vi "FGV_MG_Voltage_PCC.vi"(6 "Buffer Size":i32=10000, 7 "Command":T1, 8 "error in (no error)":errorcluster, 11 "Vabc":sgl[](array[numeric])) -> (0 "error out":errorcluster, 3 "Buffer":sgl[][](array[numeric]), 5 "Buffer Index":i32)   [LabVIEW 2015]
uses:
  Data_Queue_Command.ctl
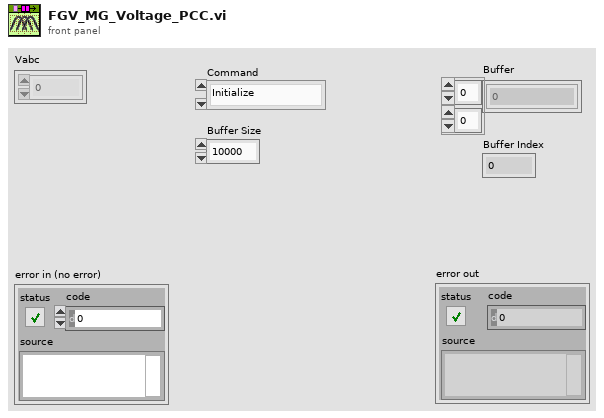
[diagram p1: front panel]
types:
  T1 = typedef "Data_Queue_Command.ctl" = enum16{"Initialize", "Write Sample", "Pull Array", "Close"}
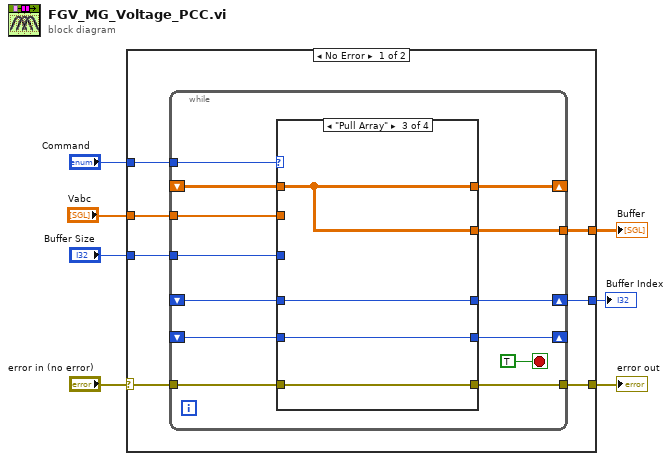
[diagram p0: block diagram]
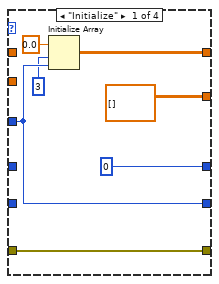
[diagram p2: hidden frame]
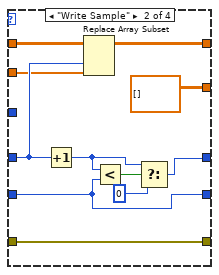
[diagram p3: hidden frame]
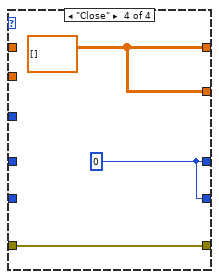
[diagram p4: hidden frame]
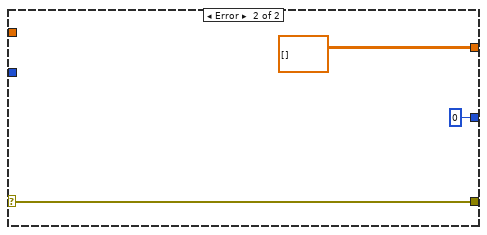
[diagram p5: hidden frame]
diagram:
  n1 = case shown="No Error" "error in (no error)" {
    selector: "error in (no error)" -> [w10 w55]
    tunnel: [w9 w55] -> w6
    tunnel: "Command" -> [w14 _]
    tunnel: "Buffer Size" -> [w13 _]
    tunnel: "Vabc" -> [w12 _]
    tunnel: [w11 sgl[][] []] -> w3
    tunnel: [w8 0 ("f")] -> w1
    frame No Error {
      n2 = while {
        tunnel: w14 -> [w26]
        tunnel: w13 -> [w25]
        tunnel: w12 -> [w24]
        shift-right: [w23] -> _
        shift-left: _ -> [w22]
        shift-right: [w21] -> _
        shift-left: _ -> [w20]
        shift-right: [w19] -> w8
        shift-left: _ -> [w18]
        tunnel: [w17] -> w11
        tunnel: w10 -> [w16]
        tunnel: [w15] -> w9
        stop <- TRUE stop-if-true
        n3 = case shown="\"Pull Array\"" w26 {
          tunnel: w25 -> [w29 _ _ _]
          tunnel: w24 -> [_ w35 _ _]
          tunnel: [w34 w40 w47 w52] -> w23
          tunnel: w22 -> [_ w45 w47 _]
          tunnel: [w29 w39 w48 w51] -> w21
          tunnel: w20 -> [_ w39 w48 _]
          tunnel: [0 ("Buffer Index") w41 w49 w51] -> w19
          tunnel: w18 -> [_ w36 w49 _]
          tunnel: [sgl[][] [] sgl[][] [] w47 w52] -> w17
          tunnel: w16 -> [w31 w37 w46 w50]
          tunnel: [w31 w37 w46 w50] -> w15
          frame "Initialize" {
            n4 = Initialize Array(sgl 0.0 ("element"), 3 ("dimension size"), w29) -> (w34:sgl[][])
          }
          frame "Write Sample" {
            n5 = Increment(x=w36) -> (x+1=w43:i32)
            n6 = Replace Array Subset(array=w45, new element=w35, index (col)=w36) -> (w40:sgl[][])  [unwired: 1 in]
            n7 = Less?(x=w43, y=w39) -> (x < y?=w44:bool)
            n8 = Select(t=w43, s=w44, f=0) -> (s? t:f=w41:i32)
          }
          frame "Pull Array" {
          }
          frame "Close" {
            w51 = 0 ("f")
            w52 = sgl[][] []
          }
        }
      }
    }
    frame Error {
    }
  }
  "Buffer" <- w3
  "error out" <- w6
  "Buffer Index" <- w1
